vi "Float.vi"() -> (0 "error out":errorcluster, 3 "Passed?":bool)   [LabVIEW 2009]
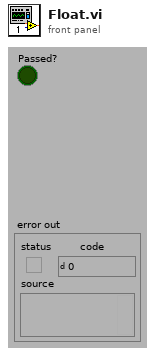
[diagram p1: front panel]
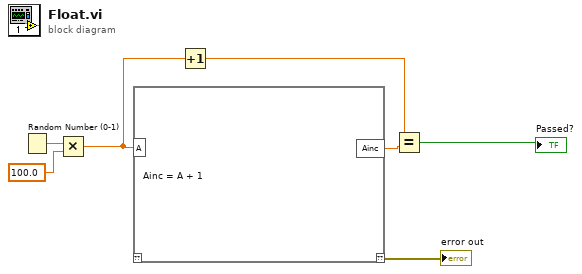
[diagram p0: block diagram]
diagram:
  n1 = Random Number (0-1)() -> (number: 0 to 1=w6:dbl)
  n2 = Multiply(x=w6, y=100.0) -> (x*y=w1:dbl)
  n3 = script code="Ainc = A + 1"("A"=w1) -> ("??"=→"error out":errorcluster, "Ainc"=w4:dbl)  [unwired: 1 in]
  n4 = Increment(x=w1) -> (x+1=w3:dbl)
  n5 = Equal?(x=w3, y=w4) -> (x = y?=→"Passed?":bool)
